vi "Check AIP buttons.vi"(8 "error in (no error)":errorcluster, 11 "RDS Local Remote Actor in":refnum<class "RDS Local Remote Actor.lvclass">) -> (0 "error out":errorcluster, 3 "RDS Local Remote Actor out":refnum<class "RDS Local Remote Actor.lvclass">)   [LabVIEW 2015, in "RDS Local Remote Actor.lvlib" / "RDS Local Remote Actor.lvclass"]
uses:
  RDS Local Remote Actor.lvclass
  RDS Local Remote Actor.lvclass/RDS Local Remote Actor.ctl
  Libraries/RDS Framework/RDS Message Class/AIP Command Control.ctl
  RDS Parent Actor/RDS Parent Actor/RDS Parent Actor.lvclass
  AIP Instrument/AIP Instrument.lvlib
  Libraries/RDS Child Messages/RDS Child Messages.lvlib
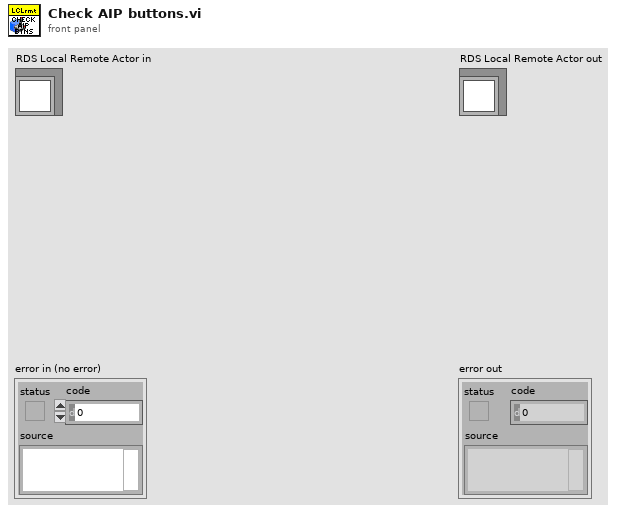
[diagram p1: front panel]
types:
  T1 = typedef "RDS Child Messages.lvlib/AIP Command Control.ctl" = enum16{"Stow", "Deploy", "Stop", "Validate Sensors", "Jog Deploy FP", "Jog Stow FP", "Jog Deploy FS", "Jog Stow FS", "Jog Deploy AP", "Jog Stow AP", "Jog Deploy AS", "Jog Stow AS", "Deploy FP", "Deploy FS", "Deploy AP", "Deploy AS", "Stow FP", "Stow FS", "Stow AP", "Stow AS"}
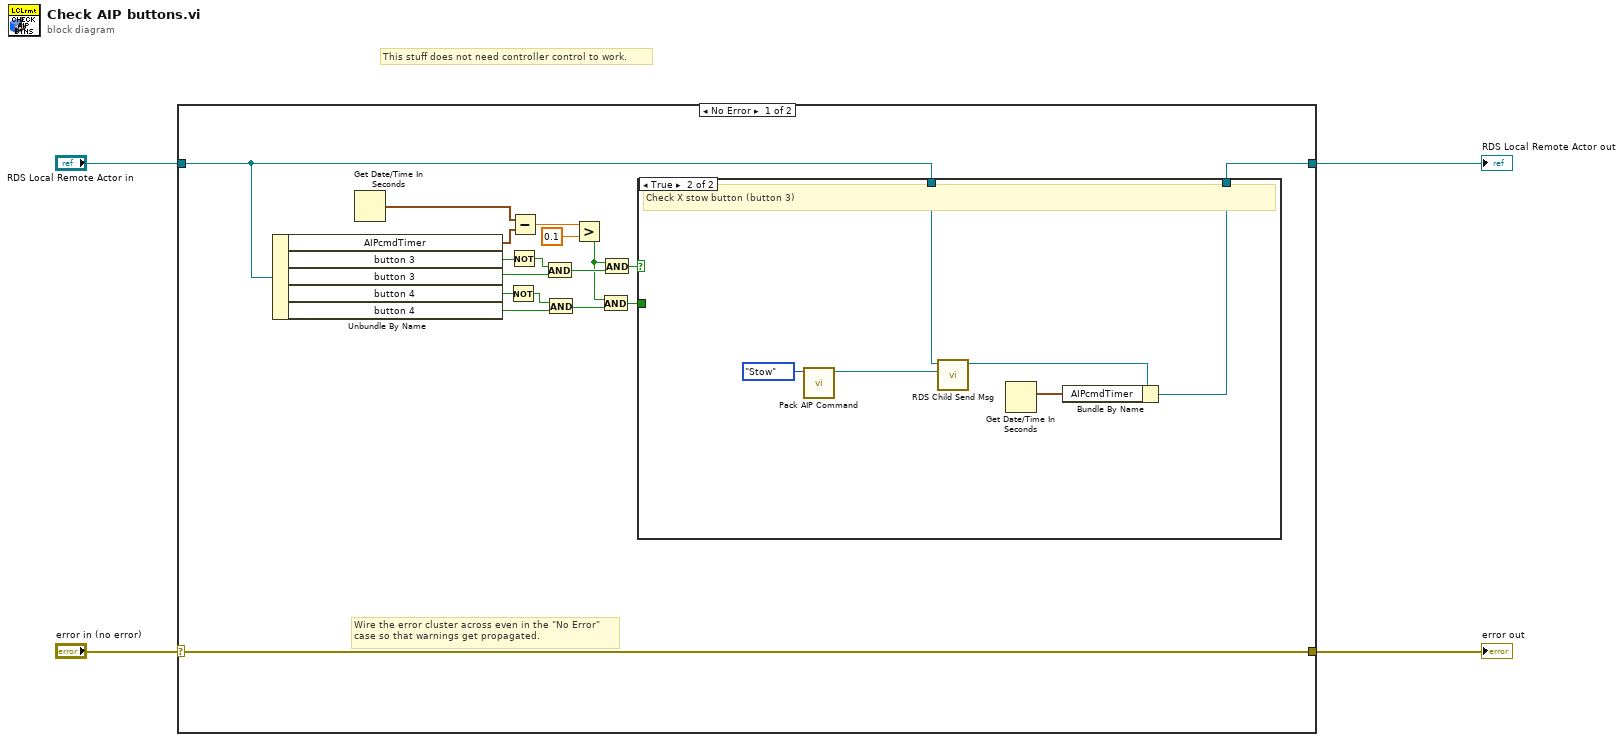
[diagram p0: block diagram]
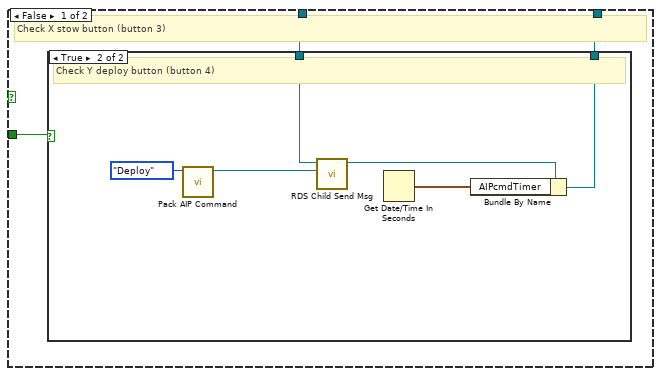
[diagram p2: hidden frame]
diagram:
  # "This stuff does not need controller control to work."
  n1 = case shown="No Error" "error in (no error)" {
    selector: "error in (no error)" -> [w22 w40]
    tunnel: [w22 w40] -> w3
    tunnel: [w5 w39] -> w1
    tunnel: "RDS Local Remote Actor in" -> [w6 w39]
    frame No Error {
      # "Wire the error cluster across even in the \"No Error\"\ncase so that warnings get propagated."
      n2 = Unbundle By Name(w6) -> ("AIPcmdTimer"=w16:timestamp, "button 3"=w21:bool, "button 3"=w19:bool, "button 4"=w12:bool, "button 4"=w10:bool)
      n3 = Get Date/Time In Seconds() -> (seconds since 1Jan1904=w15:timestamp)
      n4 = Not(x=w12) -> (.not. x?=w11:bool)
      n5 = Not(x=w21) -> (.not. x?=w20:bool)
      n6 = Subtract(x=w15, y=w16) -> (x-y=w14:dbl)
      n7 = And(x=w20, y=w19) -> (x .and. y?=w18:bool)
      n8 = And(x=w11, y=w10) -> (x .and. y?=w8:bool)
      n9 = Greater?(x=w14, y=0.1) -> (0:w9:bool)
      n10 = And(x=w9, y=w8) -> (x .and. y?=w7:bool)
      n11 = And(x=w9, y=w18) -> (x .and. y?=w17:bool)
      n12 = case shown="True" w17 {
        tunnel: w6 -> [w24 w38]
        tunnel: w7 -> [w25 _]
        tunnel: [w23 w34] -> w5
        frame False {
          # "Check X stow button (button 3)"
          n13 = case shown="True" w25 {
            tunnel: w24 -> [w26 w30]
            tunnel: [w26 w27] -> w23
            frame False {
            }
            frame True {
              # "Check Y deploy button (button 4)"
              n14 = call "Pack AIP Command.vi"("AIP Command"=AIP_Command_Control."Deploy") -> ("AIP Deploy Command out"=w32:refnum<class "AIP Command.lvclass">)  [unwired: 10 in]
              n15 = call "RDS Child Send Msg.vi"("RDS Message"=w32, "RDS Parent Actor in"=w30) -> ("RDS Parent Actor out"=w29:refnum<class "RDS Local Remote Actor.lvclass">)  [unwired: 8 in, 1 out]
              n16 = Get Date/Time In Seconds() -> (seconds since 1Jan1904=w28:timestamp)
              n17 = Bundle By Name(cluster=w29, "AIPcmdTimer"=w28) -> (w27:refnum<class "RDS Local Remote Actor.lvclass">)
            }
          }
        }
        frame True {
          # "Check X stow button (button 3)"
          n18 = call "Pack AIP Command.vi"("AIP Command"=AIP_Command_Control."Stow") -> ("AIP Deploy Command out"=w37:refnum<class "AIP Command.lvclass">)  [unwired: 10 in]
          n19 = call "RDS Child Send Msg.vi"("RDS Message"=w37, "RDS Parent Actor in"=w38) -> ("RDS Parent Actor out"=w35:refnum<class "RDS Local Remote Actor.lvclass">)  [unwired: 8 in, 1 out]
          n20 = Get Date/Time In Seconds() -> (seconds since 1Jan1904=w33:timestamp)
          n21 = Bundle By Name(cluster=w35, "AIPcmdTimer"=w33) -> (w34:refnum<class "RDS Local Remote Actor.lvclass">)
        }
      }
    }
    frame Error {
    }
  }
  "error out" <- w3
  "RDS Local Remote Actor out" <- w1
